vi "fgv_ctrl-refs-arr-1.vi"(7 "cmd":enum16{"write", "read"}(ring), 11 "ctrl-refs":refnum<vi>[](array[refnum])) -> (3 "ctrl-refs_out":refnum<vi>[](array[refnum]))   [LabVIEW 2019]
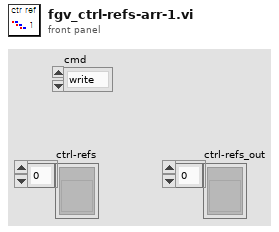
[diagram p1: front panel]
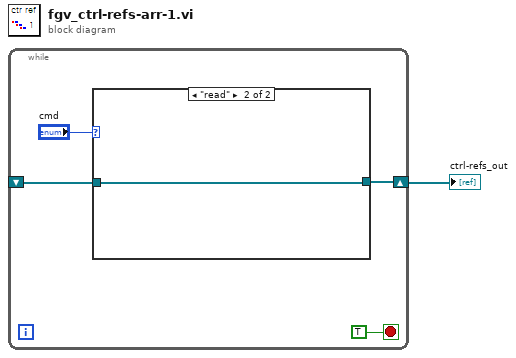
[diagram p0: block diagram]
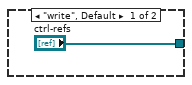
[diagram p2: hidden frame]
diagram:
  n1 = while {
    shift-right: [w3] -> w1
    shift-left: _ -> [w2]
    stop <- TRUE stop-if-true
    n2 = case shown="\"read\"" "cmd" {
      tunnel: ["ctrl-refs" w7] -> w3
      tunnel: w2 -> [_ w7]
      frame "write", Default {
      }
      frame "read" {
      }
    }
  }
  "ctrl-refs_out" <- w1
